vi "Test-DotNet-StatusMonitoring.vi"() -> ()   [LabVIEW 2013, in "HardwareCharacterization.lvlib" / "HC-SM1000.lvclass"]
uses:
  HC-SM1000.lvclass
  DOTNET-settings.ctl
  Device-identification.ctl
  Status-information.ctl
  EC1000_DOTNET/getBroadcastData-status.vi
panel:
  out "Array":i16[][](array[numeric])
  in  "Period":u32=500
  out "Graph":i16[][](graph)
  in  "Stop":bool
  out "serverList iterator":i32
  out "Status information":T1
  in  "Device index":i32
  out "piServerCount":i32
  out "Device identifiers":T2[](array[typedef])
  in  "DOTNET settings":T3={"Target IP"="128.178.146.163", "Target broadcast port"=11000, "Target communication port"=12200, "clientID"=-1, "Broadcast IP"="224.168.100.2", "Servercount"=-1, "Device IDs"=[]}
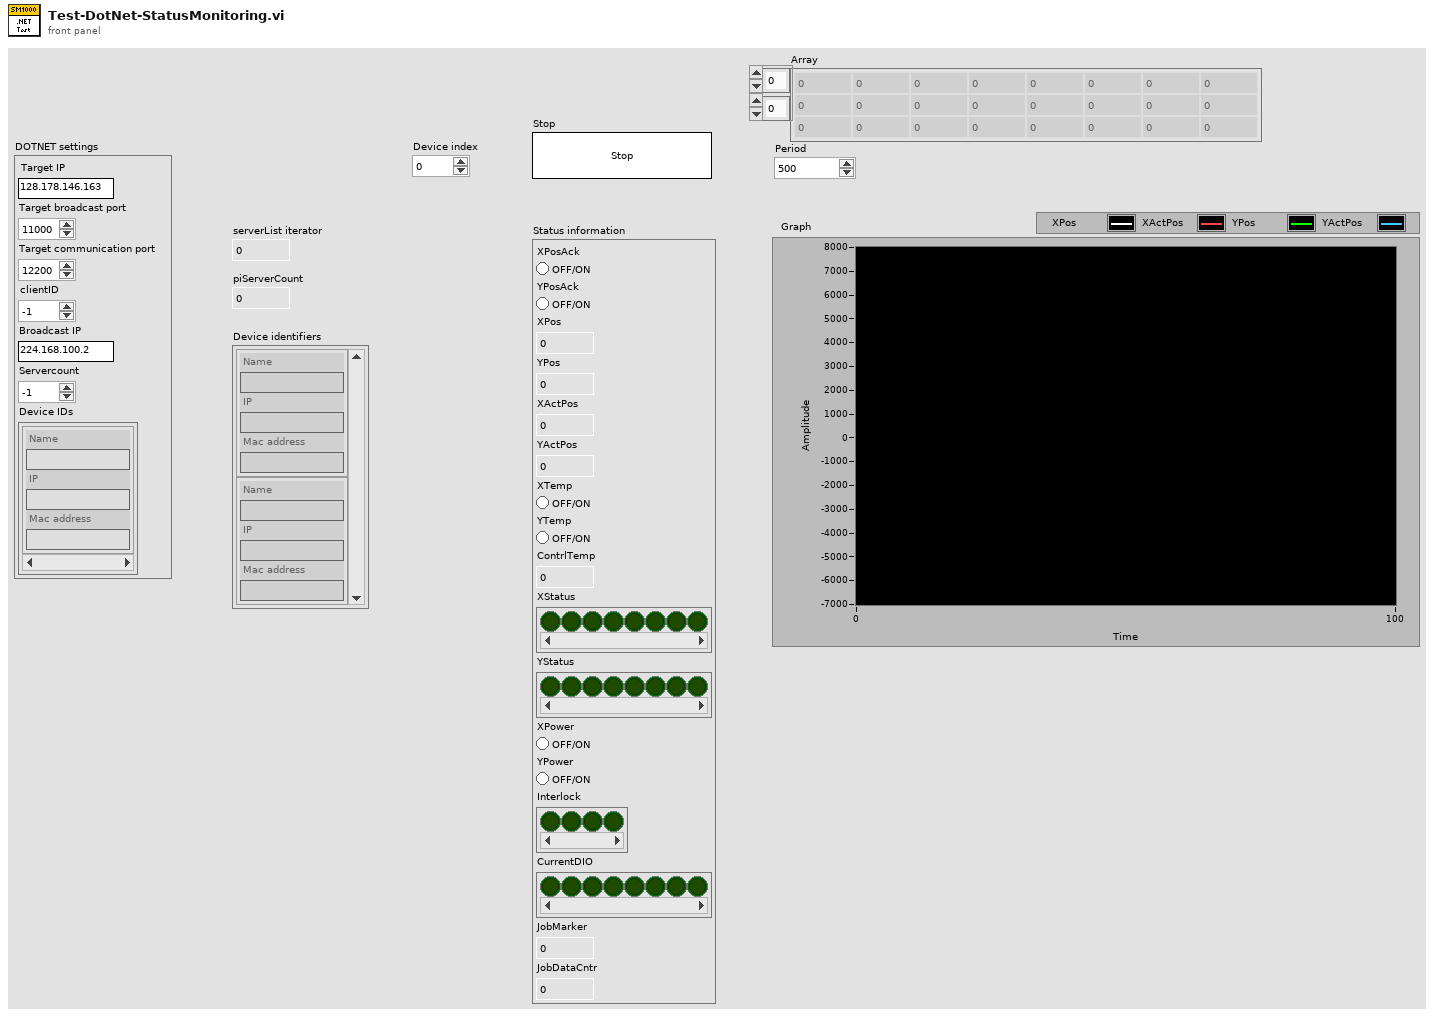
[diagram p1: front panel]
types:
  T1 = typedef "HardwareCharacterization.lvlib/HC-SM1000.lvclass/Status-information.ctl" = cluster{"XPosAck":bool, "YPosAck":bool, "XPos":i16, "YPos":i16, "XActPos":i16, "YActPos":i16, "XTemp":bool, "YTemp":bool, "ContrlTemp":i16, "XStatus":bool[], "YStatus":bool[], "XPower":bool, "YPower":bool, "Interlock":bool[], "CurrentDIO":bool[], "JobMarker":u16, "JobDataCntr":u32}
  T2 = typedef "HardwareCharacterization.lvlib/HC-SM1000.lvclass/Device-identification.ctl" = cluster{"Name":string, "IP":string, "Mac address":string}
  T3 = typedef "HardwareCharacterization.lvlib/HC-SM1000.lvclass/DOTNET-settings.ctl" = cluster{"Target IP":string, "Target broadcast port":i32, "Target communication port":i32, "clientID":i32, "Broadcast IP":string, "Servercount":i32, "Device IDs":T2[]}
  T4 = typedef "HardwareCharacterization.lvlib/HC-SM1000.lvclass/Object-reference.ctl" = refnum<data-value>
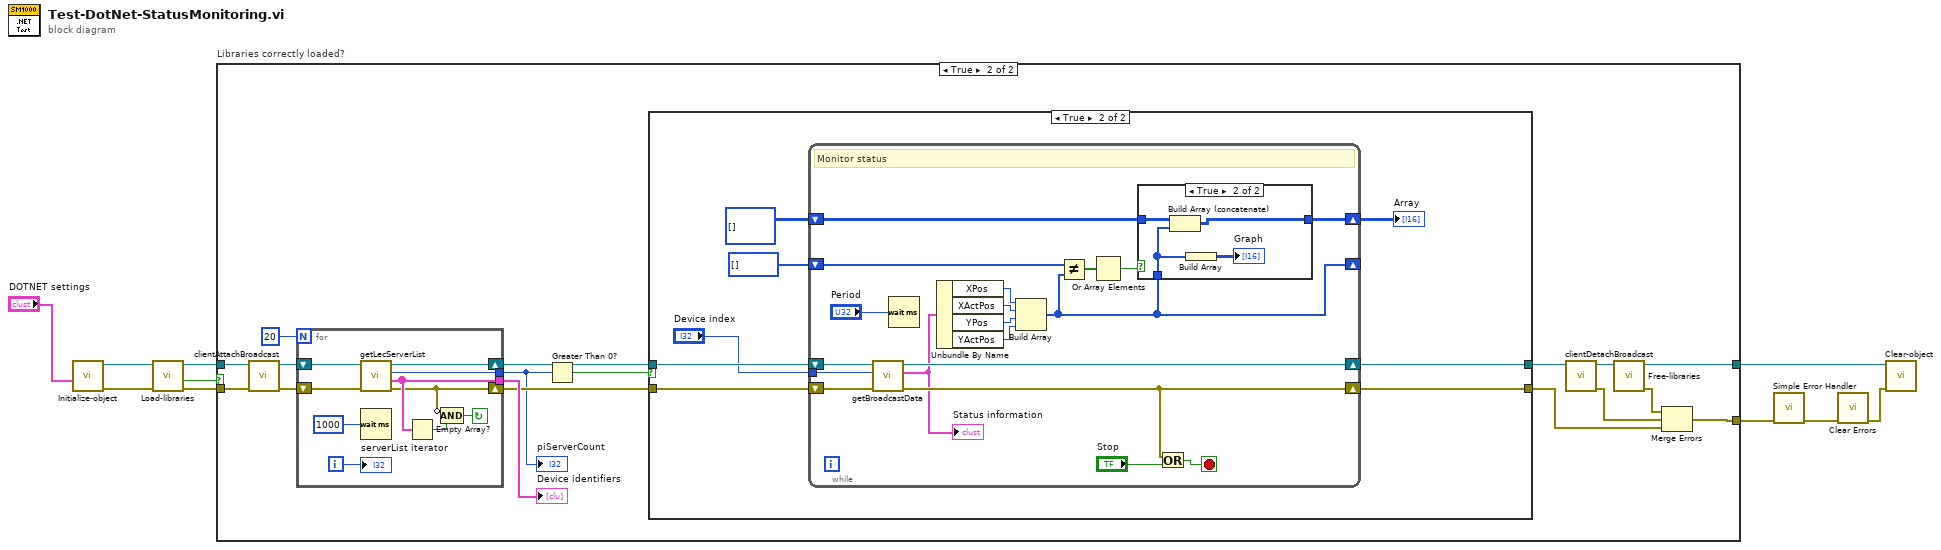
[diagram p0: block diagram]
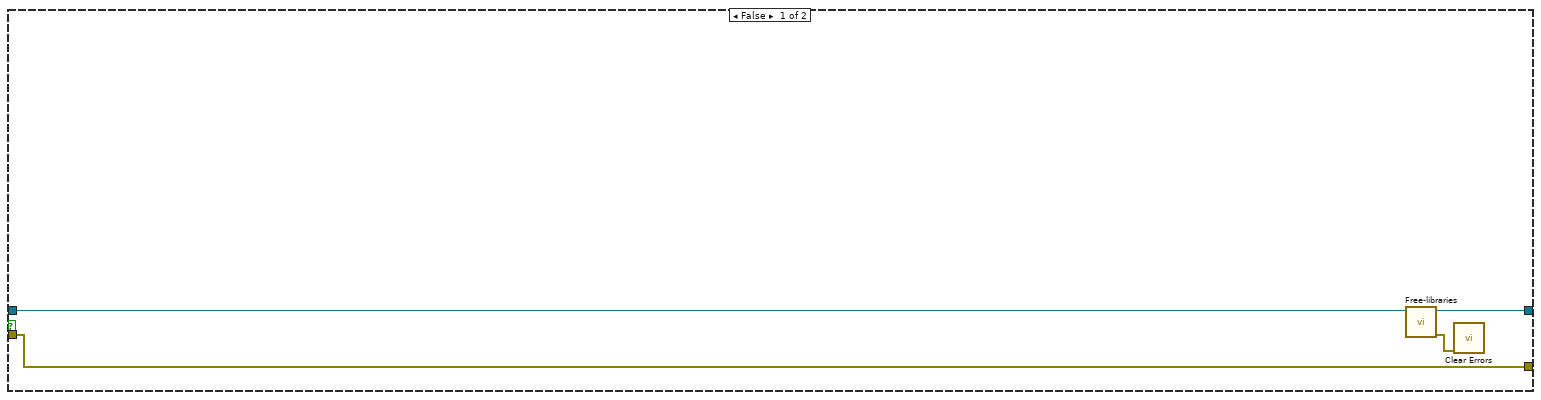
[diagram p2: hidden frame]
diagram:
  n1 = call "Initialize-object.vi"("DOTNET settings"="DOTNET settings") -> ("error out"=w8:errorcluster, "SM1000-control out"=w9:T4)  [unwired: 9 in]
  n2 = call "Load-libraries.vi"("error in (no error)"=w8, "SM1000-control in"=w9) -> ("error out"=w5:errorcluster, "Loaded?"=w7:bool, "SM1000-control out"=w6:T4)  [unwired: 7 in]
  n3 = case "Libraries correctly loaded?" shown="True" w7 {
    tunnel: w6 -> [w13 w28]
    tunnel: w5 -> [w14 w27]
    tunnel: [w14 w30] -> w3
    tunnel: [w12 w29] -> w1
    frame False {
      n4 = call "Free-libraries.vi"("SM1000-control in"=w13) -> ("error out"=w11:errorcluster, "SM1000-control out"=w12:T4)  [unwired: 8 in, 1 out]
      n5 = call <vilib>:"Clear Errors.vi"("error in (no error)"=w11) -> ()  [unwired: 6 in, 1 out]
    }
    frame True {
      n6 = call "clientAttachBroadcast.vi"("error in (no error)"=w27, "SM1000-control in"=w28) -> ("error out"=w23:errorcluster, "SM1000-control out"=w24:T4)  [unwired: 7 in, 1 out]
      n7 = for {
        N: 20 -> [_]
        tunnel: [w70] -> w22
        tunnel: [w73] -> w16
        shift-right: [w72] -> w18
        shift-left: w24 -> [w75]
        shift-right: [w67] -> w17
        shift-left: w23 -> [w74]
        i -> [w69]
        stop <- w66 continue-if-true
        n8 = call "getLecServerList.vi"("error in (no error)"=w74, "SM1000-control in"=w75) -> ("error out"=w67:errorcluster, "Device identifiers"=w70:T2[], "piServerCount"=w73:i32, "SM1000-control out"=w72:T4)  [unwired: 6 in]
        n9 = Wait (ms)(milliseconds to wait=u32 1000) -> ()  [unwired: 1 out]
        n10 = Empty Array?(array=w70) -> (empty?=w68:bool)
        n11 = Compound Arithmetic op=AND(invert w67, w68) -> (w66:bool)
        "serverList iterator" <- w69
      }
      "Device identifiers" <- w22
      "piServerCount" <- w16
      n12 = Greater Than 0?(x=w16) -> (x > 0?=w15:bool)
      n13 = case shown="True" w15 {
        tunnel: [w32 w37] -> w20
        tunnel: [w33 w38] -> w19
        tunnel: w18 -> [w33 w41]
        tunnel: w17 -> [w32 w40]
        frame False {
        }
        frame True {
          n14 = while {
            tunnel: "Device index" -> [w58]
            shift-right: [w57] -> w38
            shift-left: w41 -> [w60]
            shift-right: [w54] -> w37
            shift-left: w40 -> [w59]
            shift-right: [w43] -> _
            shift-left: i16[] [] ("appended array") -> [w47]
            shift-right: [w42] -> w34
            shift-left: i16[][] [] ("appended array") -> [w44]
            stop <- w56 stop-if-true
            # "Monitor status"
            n15 = call-poly "getBroadcastData.vi"("error in (no error)"=w59, "Device index"=w58, "SM1000-control in"=w60) -> ("error out"=w54:errorcluster, "Status information"=w53:T1, "SM1000-control out"=w57:T4)  [unwired: 6 in]
            "Status information" <- w53
            n16 = Wait (ms)(milliseconds to wait="Period") -> ()  [unwired: 1 out]
            n17 = Unbundle By Name(w53) -> ("XPos"=w50:i16, "XActPos"=w51:i16, "YPos"=w49:i16, "YActPos"=w48:i16)
            n18 = Build Array(w50, w51, w49, w48) -> (w43:i16[])
            n19 = Not Equal?(x=w47, y=w43) -> (x != y?=w46:bool[])
            n20 = Or Array Elements(Boolean array=w46) -> (logical OR=w45:bool)
            n21 = case shown="True" w45 {
              tunnel: w44 -> [w61 w65]
              tunnel: w43 -> [_ w62]
              tunnel: [w61 w64] -> w42
              frame False {
              }
              frame True {
                n22 = Build Array (concatenate)(w65, w62) -> (w64:i16[][])
                n23 = Build Array(w62) -> (→"Graph":i16[][])
              }
            }
            n24 = Or(x=w54, y="Stop") -> (x .or. y?=w56:bool)
          }
          "Array" <- w34
        }
      }
      n25 = call "clientDetachBroadcast.vi"("SM1000-control in"=w19) -> ("error out"=w25:errorcluster, "SM1000-control out"=w26:T4)  [unwired: 9 in]
      n26 = call "Free-libraries.vi"("SM1000-control in"=w26) -> ("error out"=w31:errorcluster, "SM1000-control out"=w29:T4)  [unwired: 8 in, 1 out]
      n27 = Merge Errors(w31, w25, w20) -> (w30:errorcluster)
    }
  }
  n28 = call <vilib>:"Simple Error Handler.vi"("error in (no error)"=w3) -> ("error out"=w4:errorcluster)  [unwired: 4 in, 4 out]
  n29 = call <vilib>:"Clear Errors.vi"("error in (no error)"=w4) -> ("error out"=w2:errorcluster)  [unwired: 6 in]
  n30 = call "Clear-object.vi"("error in (no error)"=w2, "SM1000-control"=w1) -> ()  [unwired: 8 in, 2 out]
